vi "Write Raw Data.vi"(8 "error in (no error)":errorcluster, 9 "Raw Data":u64[](array[numeric]), 10 "Parameters":string[](array[string]), 11 "1553 Component in":refnum<class "1553 Component.lvclass">) -> (0 "error out":errorcluster, 3 "1553 Component out":refnum<class "1553 Component.lvclass">)   [LabVIEW 2020, in "BCI-1553 API.lvlib" / "1553 Component.lvclass"]
doc: "Writes new unscaled data to a set of configured parameters for this component."
uses:
  1553 Component.lvclass
  1553 Component.lvclass/1553 Component.ctl
  1553 SubComponent/1553 SubComponent.lvclass
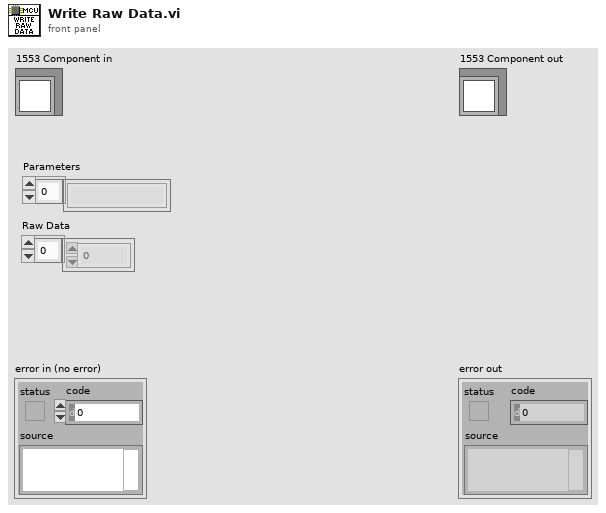
[diagram p1: front panel]
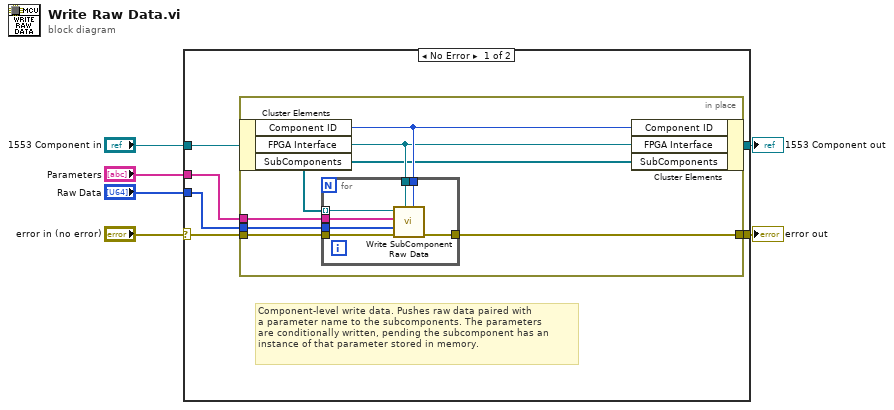
[diagram p0: block diagram]
diagram:
  n1 = case shown="No Error" "error in (no error)" {
    selector: "error in (no error)" -> [w11 w27]
    tunnel: [w10 w28] -> w3
    tunnel: "1553 Component in" -> [w12 w28]
    tunnel: "Parameters" -> [w9 _]
    tunnel: "Raw Data" -> [w8 _]
    tunnel: [w7 w27] -> w4
    frame No Error {
      # "Component-level write data. Pushes raw data paired with\na parameter name to the subcomponents. The parameters\nare conditionally written, pending the subcomponent has an\ninstance of that parameter stored in memory."
      n2 = in-place {
        in-place-border: w11 -> [w17]
        in-place-border: w9 -> [w16]
        in-place-border: w8 -> [w15]
        in-place-border: [w13] -> w7
        n3 = in-place-cluster #1(w12) -> ("Component ID"=w19:u8, "FPGA Interface"=w18:refnum<class "FPGA Interface.lvclass">, "SubComponents"=w14:refnum<class "1553 SubComponent.lvclass">[])
        n4 = for {
          tunnel: w14 -> [w24] mode=indexing
          tunnel: w19 -> [w25]
          tunnel: w18 -> [w26]
          tunnel: w17 -> [w23]
          tunnel: w16 -> [w21]
          tunnel: w15 -> [w20]
          tunnel: [w22] -> w13
          n5 = call-dynamic "Write SubComponent Raw Data.vi"("Component ID"=w25, "FPGA Interface"=w26, "error in (no error)"=w23, "Raw Data"=w20, "Parameters"=w21, "1553 SubComponent in"=w24) -> ("error out"=w22:errorcluster)  [unwired: 5 in]
        }
        n6 = in-place-cluster #1("Component ID"=w19, "FPGA Interface"=w18, "SubComponents"=w14) -> (w10:refnum<class "1553 Component.lvclass">)
      }
    }
    frame Error {
    }
  }
  "error out" <- w4
  "1553 Component out" <- w3
